vi "KTBT32工位修改模通讯协议.vi"(0 "开关控制":bool[](array[boolean]), 5 "通道号":u8 max=31, 9 "接收指令":string, 11 "error in":errorcluster) -> (4 "发送指令":string, 10 "Array":string[](array[string]), 15 "error out":errorcluster)   [LabVIEW 2016]
panel:
  out "element":bool
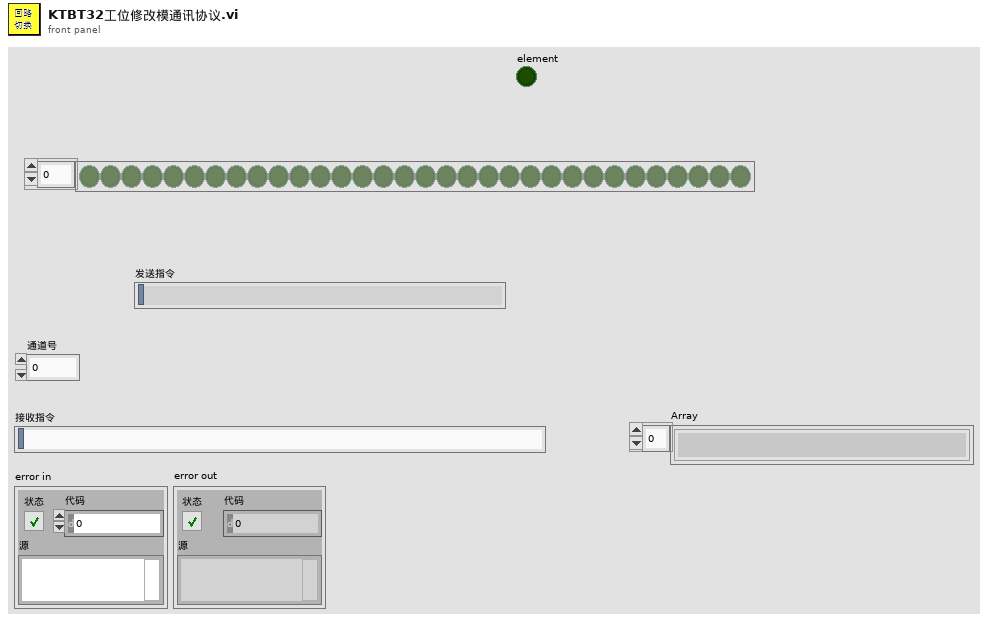
[diagram p1: front panel]
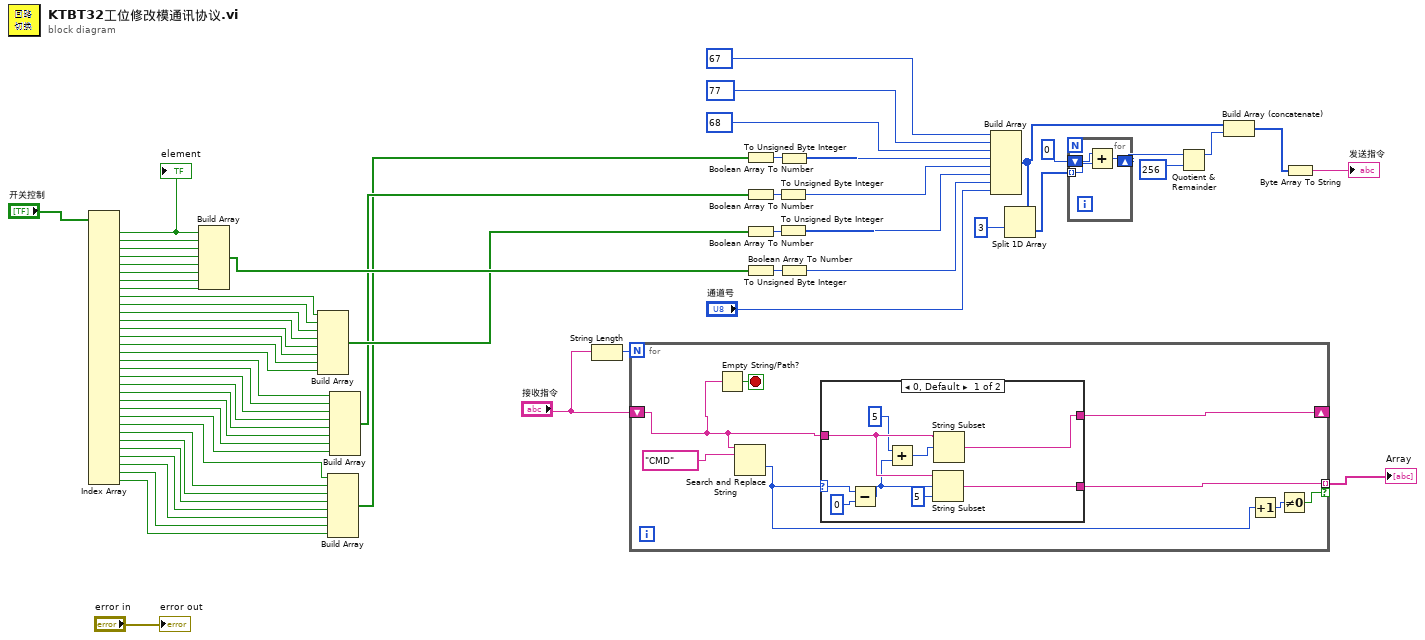
[diagram p0: block diagram]
diagram:
  n1 = Index Array(array="开关控制") -> (element #1=w36:bool, element #2=w35:bool, element #3=w34:bool, element #4=w33:bool, element #5=w32:bool, element #6=w31:bool, element #7=w30:bool, element #8=w29:bool, element #9=w28:bool, element #10=w27:bool, element #11=w26:bool, element #12=w25:bool, element #13=w24:bool, element #14=w23:bool, element #15=w22:bool, element #16=w21:bool, element #17=w20:bool, element #18=w19:bool, element #19=w18:bool, element #20=w17:bool, element #21=w16:bool, element #22=w15:bool, element #23=w14:bool, element #24=w13:bool, element #25=w12:bool, element #26=w11:bool, element #27=w10:bool, element #28=w9:bool, element #29=w8:bool, element #30=w7:bool, element #31=w6:bool, element #32=w5:bool)  [unwired: 32 in]
  "element" <- w36
  n2 = Build Array(w36, w35, w34, w33, w32, w31, w30, w29) -> (w4:bool[])
  n3 = Build Array(w28, w27, w26, w25, w24, w23, w22, w21) -> (w3:bool[])
  n4 = Build Array(w12, w11, w10, w9, w8, w7, w6, w5) -> (w1:bool[])
  n5 = Build Array(w20, w19, w18, w17, w16, w15, w14, w13) -> (w2:bool[])
  n6 = String Length(string="接收指令") -> (length=w44:i32)
  n7 = for {
    N: w44 -> [_]
    shift-right: [w68] -> _
    shift-left: "接收指令" -> [w66]
    tunnel: [w70] -> w43 mode=indexing if=w65
    stop <- w69 stop-if-true
    n8 = Empty String/Path?(string/path=w66) -> (empty?=w69:bool)
    n9 = Search and Replace String(input string=w66, search string="CMD" ("下发指令")) -> (offset past replacement=w63:i32)  [unwired: 6 in, 3 out]
    n10 = case shown="0, Default" w63 {
      selector: w63 -> [w73 _]
      tunnel: w66 -> [w79 _]
      tunnel: [w75 _] -> w68
      tunnel: [w76 _] -> w70
      frame 0, Default {
        n11 = Subtract(x=w73, y=0) -> (x-y=w72:i32)
        n12 = Add(x=5 ("offset past match"), y=w72) -> (x+y=w74:i32)
        n13 = String Subset(string=w79, offset (0)=w72, length (rest)=5 ("offset past match")) -> (substring=w76:string)
        n14 = String Subset(string=w79, offset (0)=w74) -> (substring=w75:string)  [unwired: 1 in]
      }
      frame -1 {
      }
    }
    n15 = Increment(x=w63) -> (x+1=w64:i32)
    n16 = Not Equal To 0?(x=w64) -> (x != 0?=w65:bool)
  }
  "Array" <- w43
  n17 = Boolean Array To Number(Boolean array=w1) -> (number=w58:u32)
  n18 = Boolean Array To Number(Boolean array=w2) -> (number=w56:u32)
  n19 = Boolean Array To Number(Boolean array=w3) -> (number=w54:u32)
  n20 = Boolean Array To Number(Boolean array=w4) -> (number=w52:u32)
  n21 = To Unsigned Byte Integer(number=w56) -> (unsigned 8bit integer=w55:u8)
  n22 = To Unsigned Byte Integer(number=w54) -> (unsigned 8bit integer=w53:u8)
  n23 = To Unsigned Byte Integer(number=w58) -> (unsigned 8bit integer=w57:u8)
  n24 = To Unsigned Byte Integer(number=w52) -> (unsigned 8bit integer=w51:u8)
  n25 = Build Array(u8 67, u8 77, u8 68, w57, w55, w53, w51, "通道号") -> (w41:u8[])
  n26 = Split 1D Array(array=w41, index=3) -> (second subarray=w39:u8[])  [unwired: 1 out]
  n27 = for {
    tunnel: w39 -> [w81] mode=indexing
    shift-right: [w80] -> w48
    shift-left: 0 -> [w82]
    n28 = Add(x=w82, y=w81) -> (x+y=w80:i32)
  }
  n29 = Quotient & Remainder(x=w48, y=256) -> (x-y*floor(x/y)=w46:i32)  [unwired: 1 out]
  n30 = Build Array (concatenate)(w41, w46) -> (w45:i32[])
  n31 = Byte Array To String(unsigned byte array=w45) -> (string=→"发送指令":string)
  "error out" <- "error in"
